vi "TC01lib.vi"(10 "physical channel":string="Dev2/ai0", 11 "thermocouple type":i32(ring)=10072 items=["J"=10072, "K"=10073, "N"=10077, "R"=10082, "S"=10085, "T"=10086, "B"=10047, "E"=10055]) -> (3 "data":dbl format="%0.2f")   [LabVIEW 2012]
uses:
  <vilib>/DAQmx/read.llb/DAQmx Read.vi
  <vilib>/DAQmx/read.llb/DAQmx Read (Analog DBL 1Chan 1Samp).vi
  <vilib>/DAQmx/miscellaneous.llb/DAQmx Fill In Error Info.vi
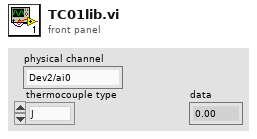
[diagram p1: front panel]
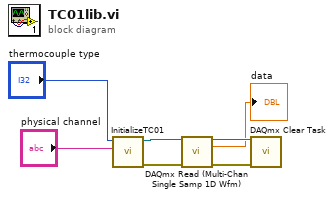
[diagram p0: block diagram]
diagram:
  n1 = call "InitializeTC01.vi"("physical channel"="physical channel", "thermocouple type"="thermocouple type") -> ("error out"=w4:errorcluster, "task out"=w5:refnum<k21>)  [unwired: 8 in]
  n2 = call-poly "DAQmx Read (Multi-Chan Single Samp 1D Wfm).vi"("task/channels in"=w5, "error in"=w4) -> ("task out"=w7:refnum<k21>, "data"=→"data":dbl, "error out"=w6:errorcluster)  [unwired: 11 out]
  n3 = call <vilib>:"DAQmx Clear Task.vi"("task in"=w7, "error in"=w6) -> ()  [unwired: 14 out]
